vi "WFRM_attribute_chart.vi"() -> ()   [LabVIEW 2019]
panel:
  in  "Y":dbl[](array[numeric]) format="%#.6g"
  out "Waveform Chart":dbl[unit][](graph)
  in  "Waveform":waveform(dbl)
  out "Waveform Graph":waveform(dbl)(graph)
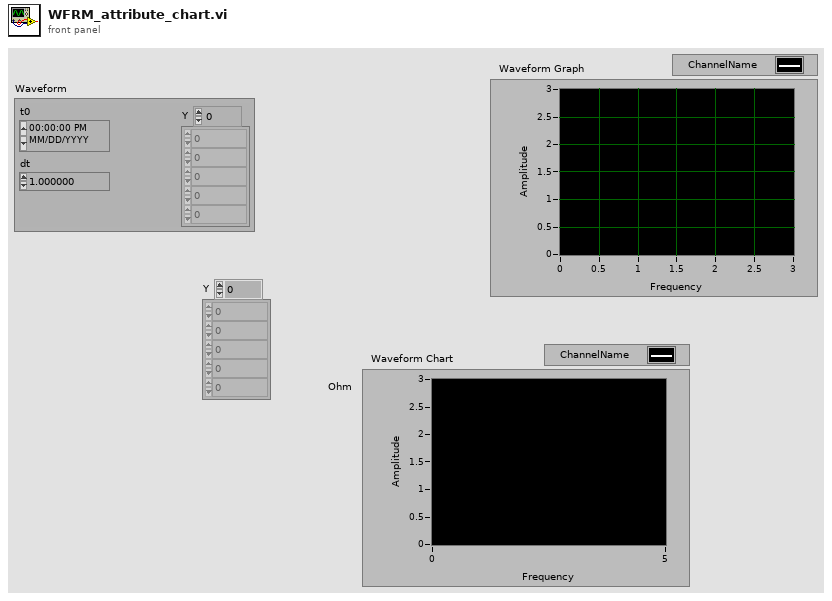
[diagram p1: front panel]
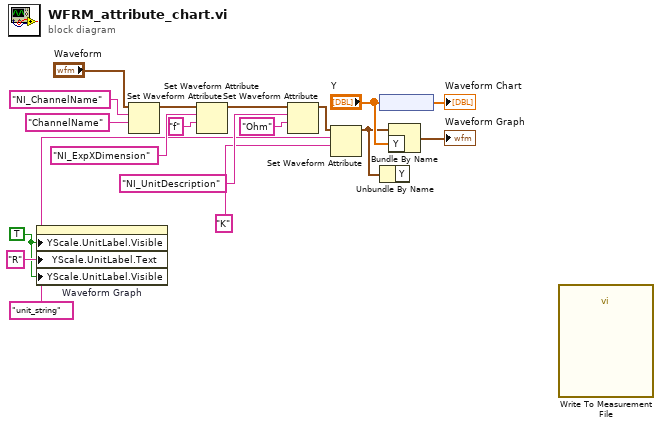
[diagram p0: block diagram]
diagram:
  w8 = TRUE ("Y Scale.Unit Label.Visible")
  n1 = property on="Waveform Graph" class="WFGraph (strict)"("YScale.UnitLabel.Visible"=w8, "YScale.UnitLabel.Text"="R" ("Y Scale.Unit Label.Text"), "YScale.UnitLabel.Visible"=w8) -> ()  [unwired: 2 in, 2 out]
  n2 = Set Waveform Attribute(5:"ChannelName" ("name"), 6:"NI_ChannelName" ("name"), 7:"Waveform") -> (3:w17:waveform(dbl))  [unwired: 1 in, 2 out]
  n3 = Set Waveform Attribute(5:"f" ("name"), 6:"NI_ExpXDimension" ("name"), 7:w17) -> (3:w12:waveform(dbl))  [unwired: 1 in, 2 out]
  n4 = Set Waveform Attribute(5:"Ohm" ("name"), 6:"NI_UnitDescription" ("name"), 7:w12) -> (3:w7:waveform(dbl))  [unwired: 1 in, 2 out]
  n5 = Set Waveform Attribute(5:"K" ("Y Scale.Unit Label.Text"), 6:"unit_string" ("name"), 7:w7) -> (3:w3:waveform(dbl))  [unwired: 1 in, 2 out]
  n6 = node("Y") -> (→"Waveform Chart":dbl[unit][])
  n7 = Unbundle By Name(w3) -> ()  [unwired: 1 out]
  n8 = Bundle By Name(cluster=w3, "Y"="Y") -> (→"Waveform Graph":waveform(dbl))
  n9 = call "Write To Measurement File"() -> ()  [unwired: 17 in, 3 out]
